vi "ke37xx Configure Math.vi"(0 "VISA Resource Name":refnum<visa-resource-name>, 5 "Enabled (True)":bool=TRUE, 7 "Operation Type (0: None)":T1(ring), 9 "Percent Constant":dbl, 11 "error in (no error)":errorcluster, 12 "Mxb Offset":dbl, 13 "Mxb Scale Factor":dbl) -> (4 "VISA Resource Name Out":refnum<visa-resource-name>, 15 "error out":errorcluster)   [LabVIEW 2009, in "Keithley 3700 Series.lvlib"]
doc: "This VI allows you to configure how math operations are performed on measurement."
uses:
  <instrlib>/Keithley 3706/Keithley 3700 Series.lvlib
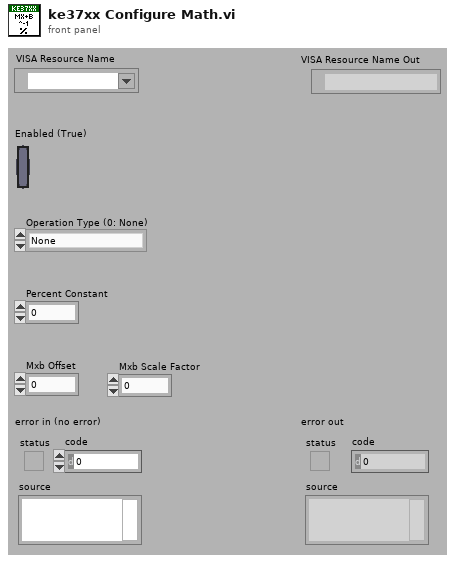
[diagram p1: front panel]
types:
  T1 = enum16{"None", "Mx + b", "Percent", "Reciprocal"}
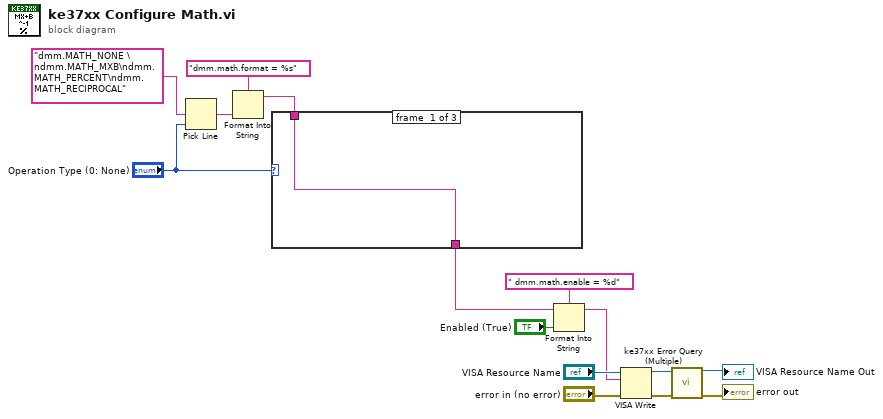
[diagram p0: block diagram]
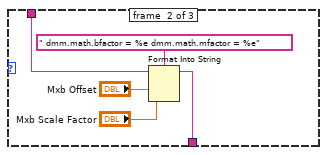
[diagram p2: hidden frame]
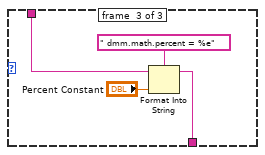
[diagram p3: hidden frame]
diagram:
  n1 = Pick Line(multi-line string="dmm.MATH_NONE \ndmm.MATH_MXB\ndmm.MATH_PERCENT\ndmm.MATH_RECIPROCAL", line index="Operation Type (0: None)") -> (output string=w7:string)  [unwired: 1 out]
  n2 = Format Into String(format string="dmm.math.format = %s" ("write buffer"), w7) -> (resulting string=w5:string)  [unwired: 2 in, 1 out]
  n3 = case shown="\"Percent\"" "Operation Type (0: None)" {
    tunnel: w5 -> [w16 w20 w24]
    tunnel: [w16 w17 w22] -> w2
    frame #0 {
    }
    frame #1 {
      n4 = Format Into String(format string=" dmm.math.bfactor = %e dmm.math.mfactor = %e" ("write buffer"), initial string=w20, "Mxb Offset", "Mxb Scale Factor") -> (resulting string=w17:string)  [unwired: 1 in, 1 out]
    }
    frame #2 {
      n5 = Format Into String(format string=" dmm.math.percent = %e" ("write buffer"), initial string=w24, "Percent Constant") -> (resulting string=w22:string)  [unwired: 1 in, 1 out]
    }
  }
  n6 = Format Into String(format string=" dmm.math.enable = %d" ("write buffer"), initial string=w2, "Enabled (True)") -> (resulting string=w1:string)  [unwired: 1 in, 1 out]
  n7 = VISA Write(VISA resource name="VISA Resource Name", write buffer=w1, error in (no error)="error in (no error)") -> (VISA resource name out=w11:refnum<visa-resource-name>, error out=w10:errorcluster)  [unwired: 1 out]
  n8 = call <instrlib>:"ke37xx Error Query (Multiple).vi"("VISA resource name"=w11, "error in (no error)"=w10) -> ("VISA resource name out"=→"VISA Resource Name Out":refnum<visa-resource-name>, "error out"=→"error out":errorcluster)  [unwired: 12 out]
